vi "Engine - Add content to Engine library.vi"(8 "error in (no error)":errorcluster, 11 "CD Wizard - Internal Data IN":T1) -> (0 "error out":errorcluster)   [LabVIEW 2015]
doc: "Add all virtual folders and VIs to the Engine library."
uses:
  TypDef/CD Wizard - Internal data.ctl
  TypDef/CD Wizard - Execution Mode.ctl
  TypDef/CD Wizard - Extra Page Name and GUID.ctl
  Constants/Constants TypDef/CD Engine lvlib.ctl
  TypDef/Add Item - Type.ctl
  Constants/CD Engine lvlib.vi
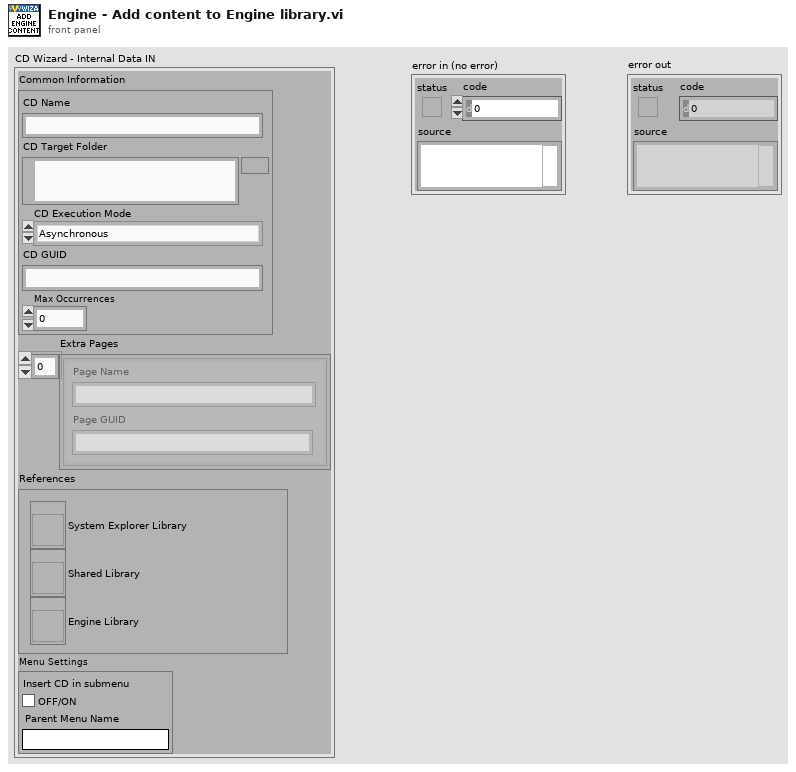
[diagram p1: front panel]
types:
  T1 = typedef "CD Wizard - Internal data.ctl" = cluster{"Common Information":cluster{"CD Name":string, "CD Target Folder":path, "CD Execution Mode":T2, "CD GUID":string, "Max Occurrences":u32}, "Extra Pages":T3[], "References":cluster{"System Explorer Library":refnum<vi>, "Shared Library":refnum<vi>, "Engine Library":refnum<vi>}, "Menu Settings":cluster{"Insert CD in submenu":bool, "Parent Menu Name":string}}
  T2 = typedef "CD Wizard - Execution Mode.ctl" = enum16{"Asynchronous", "Inline HW Interface", "Inline Model Interface", "Inline Timing and Sync", "Asynchronous Timing and Sync"}
  T3 = typedef "CD Wizard - Extra Page Name and GUID.ctl" = cluster{"Page Name":string, "Page GUID":string}
  T4 = typedef "CD Engine lvlib.ctl" = enum16{"LibraryFileName", "LibraryFolderName", "Engine.FolderName", "Engine.Init.FolderName", "Engine.Run.FolderName", "Engine.Shutdown.FolderName", "Types.FolderName", "Engine.RT Driver VI.TemplatePath", "Engine.RT Driver VI.FileName", "Engine.RTStateVariables.Name", "Engine.Async.NameExtension"}
  T5 = typedef "Add Item - Type.ctl" = string
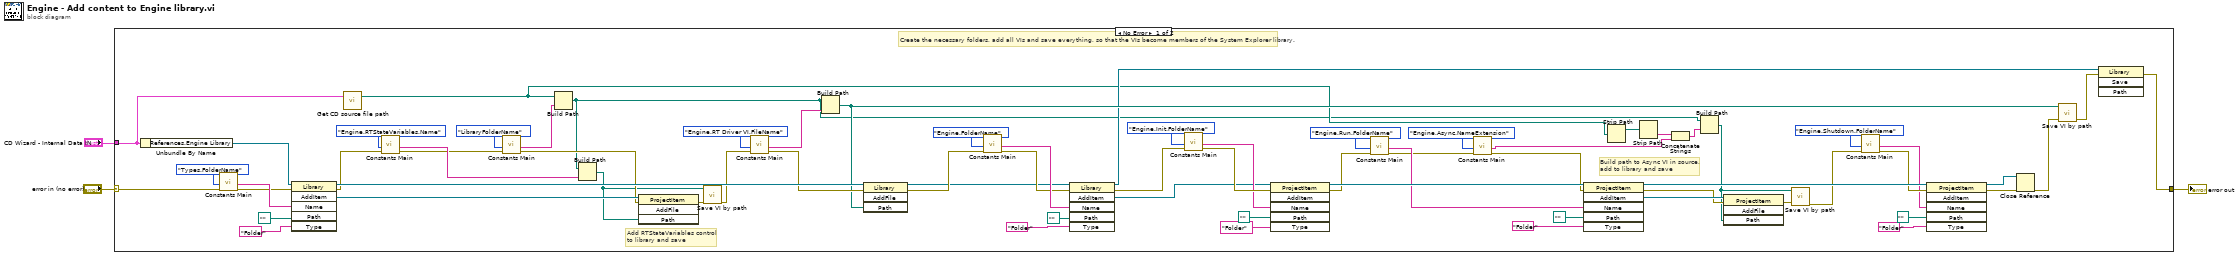
[diagram p0: block diagram]
diagram:
  n1 = case shown="No Error" "error in (no error)" {
    selector: "error in (no error)" -> [w56 w74]
    tunnel: "CD Wizard - Internal Data IN" -> [w30 _]
    tunnel: [w73 w74] -> w1
    frame No Error {
      # "Add RTStateVariables control\nto library and save"
      # "Build path to Async VI in source,\nadd to library and save"
      # "Create the necessary folders, add all VIs and save everything, so that the VIs become members of the System Explorer library."
      n2 = Unbundle By Name(w30) -> ("References.Engine Library"=w55:refnum<vi>)
      n3 = call-poly "Constants Main.vi"("error in (no error)"=w56, "Action"=CD_Engine_lvlib."Types.FolderName") -> ("error out"=w68:errorcluster, "Output"=w70:string)  [unwired: 8 in]
      n4 = invoke class="Library" method="AddItem"(reference=w55, error in=w68, "Name"=w70, "Path"=path "", "Type"=T5 "Folder" ("Add Item - Type")) -> (reference out=w63:refnum<vi>, error out=w6:errorcluster, "AddItem"=w26:refnum<vi>)  [unwired: 1 in, 3 out]
      n5 = call "Get CD source file path.vi"("CD Wizard - Internal Data"=w30) -> ("CD Source file path"=w19:path)  [unwired: 2 in]
      n6 = call-poly "Constants Main.vi"("error in (no error)"=w6, "Action"=CD_Engine_lvlib."Engine.RTStateVariables.Name") -> ("error out"=w4:errorcluster, "Output"=w5:string)  [unwired: 8 in]
      n7 = call-poly "Constants Main.vi"("error in (no error)"=w4, "Action"=CD_Engine_lvlib."LibraryFolderName") -> ("error out"=w25:errorcluster, "Output"=w59:string)  [unwired: 8 in]
      n8 = Build Path(base path=w19, name or relative path=w59) -> (appended path=w16:path)
      n9 = Build Path(base path=w16, name or relative path=w5) -> (appended path=w22:path)
      n10 = invoke class="ProjectItem" method="AddFile"(reference=w26, error in=w25, "Path"=w22) -> (error out=w24:errorcluster)  [unwired: 1 in, 3 out]
      n11 = call "Save VI by path.vi"("error in (no error)"=w24, "VI path"=w22) -> ("error out"=w23:errorcluster)  [unwired: 9 in]
      n12 = call-poly "Constants Main.vi"("error in (no error)"=w23, "Action"=CD_Engine_lvlib."Engine.RT Driver VI.FileName") -> ("error out"=w57:errorcluster, "Output"=w61:string)  [unwired: 8 in]
      n13 = Build Path(base path=w16, name or relative path=w61) -> (appended path=w33:path)
      n14 = invoke class="Library" method="AddFile"(reference=w63, error in=w57, "Path"=w33) -> (reference out=w48:refnum<vi>, error out=w50:errorcluster)  [unwired: 1 in, 2 out]
      n15 = call-poly "Constants Main.vi"("error in (no error)"=w50, "Action"=CD_Engine_lvlib."Engine.FolderName") -> ("error out"=w49:errorcluster, "Output"=w52:string)  [unwired: 8 in]
      n16 = invoke class="Library" method="AddItem"(reference=w48, error in=w49, "Name"=w52, "Path"=path "", "Type"=T5 "Folder" ("Add Item - Type")) -> (reference out=w32:refnum<vi>, error out=w45:errorcluster, "AddItem"=w47:refnum<vi>)  [unwired: 1 in, 3 out]
      n17 = call-poly "Constants Main.vi"("error in (no error)"=w45, "Action"=CD_Engine_lvlib."Engine.Init.FolderName") -> ("error out"=w66:errorcluster, "Output"=w64:string)  [unwired: 8 in]
      n18 = invoke class="ProjectItem" method="AddItem"(reference=w47, error in=w66, "Name"=w64, "Path"=path "", "Type"=T5 "Folder" ("Add Item - Type")) -> (reference out=w44:refnum<vi>, error out=w41:errorcluster)  [unwired: 1 in, 4 out]
      n19 = call-poly "Constants Main.vi"("error in (no error)"=w41, "Action"=CD_Engine_lvlib."Engine.Run.FolderName") -> ("error out"=w10:errorcluster, "Output"=w42:string)  [unwired: 8 in]
      n20 = call-poly "Constants Main.vi"("error in (no error)"=w10, "Action"=CD_Engine_lvlib."Engine.Async.NameExtension") -> ("error out"=w8:errorcluster, "Output"=w9:string)  [unwired: 8 in]
      n21 = invoke class="ProjectItem" method="AddItem"(reference=w44, error in=w8, "Name"=w42, "Path"=path "", "Type"=T5 "Folder" ("Add Item - Type")) -> (reference out=w35:refnum<vi>, error out=w15:errorcluster, "AddItem"=w18:refnum<vi>)  [unwired: 1 in, 3 out]
      n22 = Strip Path(path=w19) -> (stripped path=w21:path)  [unwired: 1 out]
      n23 = Strip Path(path=w21) -> (name=w20:string)  [unwired: 1 out]
      n24 = Concatenate Strings(w20, w9) -> (w17:string)
      n25 = Build Path(base path=w16, name or relative path=w17) -> (appended path=w13:path)
      n26 = invoke class="ProjectItem" method="AddFile"(reference=w18, error in=w15, "Path"=w13) -> (error out=w14:errorcluster)  [unwired: 1 in, 3 out]
      n27 = call "Save VI by path.vi"("error in (no error)"=w14, "VI path"=w13) -> ("error out"=w12:errorcluster)  [unwired: 9 in]
      n28 = call-poly "Constants Main.vi"("error in (no error)"=w12, "Action"=CD_Engine_lvlib."Engine.Shutdown.FolderName") -> ("error out"=w34:errorcluster, "Output"=w31:string)  [unwired: 8 in]
      n29 = invoke class="ProjectItem" method="AddItem"(reference=w35, error in=w34, "Name"=w31, "Path"=path "", "Type"=T5 "Folder" ("Add Item - Type")) -> (reference out=w27:refnum<vi>, error out=w29:errorcluster)  [unwired: 1 in, 4 out]
      n30 = Close Reference(reference=w27, error in (no error)=w29) -> (error out=w28:errorcluster)
      n31 = call "Save VI by path.vi"("error in (no error)"=w28, "VI path"=w33) -> ("error out"=w72:errorcluster)  [unwired: 9 in]
      n32 = invoke class="Library" method="Save"(reference=w32, error in=w72) -> (error out=w73:errorcluster)  [unwired: 2 in, 3 out]
    }
    frame Error {
      # "Output default values."
    }
  }
  "error out" <- w1
